vi "square_root.vi"() -> ()   [LabVIEW 2019]
panel:
  in  "stop":bool
  out "sqrt(x)":dbl
  in  "x":dbl
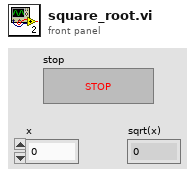
[diagram p1: front panel]
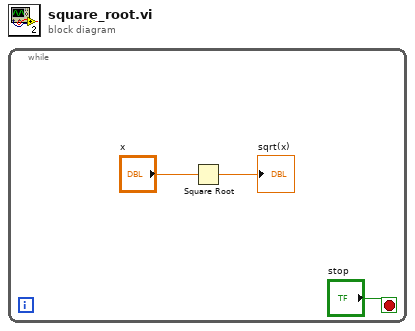
[diagram p0: block diagram]
diagram:
  n1 = while {
    stop <- "stop" stop-if-true
    n2 = Square Root(x="x") -> (sqrt(x)=→"sqrt(x)":dbl)
  }
